vi "GetLVServicerBuildSpecPath.vi"(11 "Base Path":path) -> (3 "LV Servicer Build Spec Path":path)   [LabVIEW 2019]
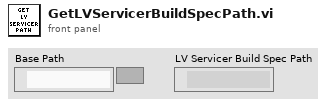
[diagram p1: front panel]
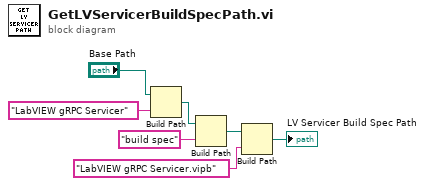
[diagram p0: block diagram]
diagram:
  n1 = Build Path(base path="Base Path", name or relative path="LabVIEW gRPC Servicer") -> (appended path=w3:path)
  n2 = Build Path(base path=w3, name or relative path="build spec") -> (appended path=w5:path)
  n3 = Build Path(base path=w5, name or relative path="LabVIEW gRPC Servicer.vipb") -> (appended path=→"LV Servicer Build Spec Path":path)
